vi "RichToFlatcif_channelcore_CreateFIFOInstanceResponse.vi"(5 "OutputClusterType":T1, 11 "InputCluster":T4) -> (3 "OutputCluster":T1)   [LabVIEW 2021, in "CIFCoreChannel_server.lvlib"]
uses:
  CIFCoreChannel_server.lvlib
  cif_channelcore_CreateFIFOInstanceResponse.ctl
  cif_channelcore_FIFOReference.ctl
  cif_common_Status.ctl
  cif_channelcore_CreateFIFOInstanceResponse_Flat.ctl
  cif_channelcore_FIFOReference_Flat.ctl
  cif_common_Status_Flat.ctl
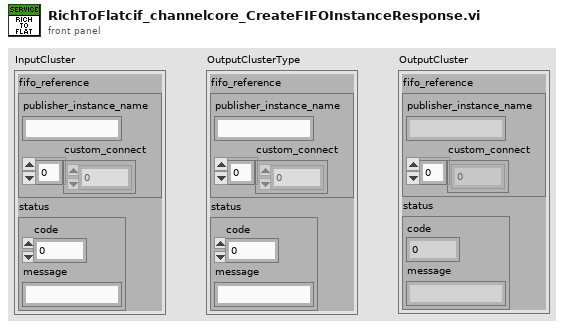
[diagram p1: front panel]
types:
  T1 = typedef "CIFCoreChannel_server.lvlib/cif_channelcore_CreateFIFOInstanceResponse_Flat.ctl" = cluster{"fifo_reference":T2, "status":T3}
  T2 = typedef "CIFCoreChannel_server.lvlib/cif_channelcore_FIFOReference_Flat.ctl" = cluster{"publisher_instance_name":string, "custom_connect":u8[]}
  T3 = typedef "CIFCoreChannel_server.lvlib/cif_common_Status_Flat.ctl" = cluster{"code":i32, "message":string}
  T4 = typedef "CIFCoreChannel_server.lvlib/cif_channelcore_CreateFIFOInstanceResponse.ctl" = cluster{"fifo_reference":T5, "status":T6}
  T5 = typedef "CIFCoreChannel_server.lvlib/cif_channelcore_FIFOReference.ctl" = cluster{"publisher_instance_name":string, "custom_connect":u8[]}
  T6 = typedef "CIFCoreChannel_server.lvlib/cif_common_Status.ctl" = cluster{"code":i32, "message":string}
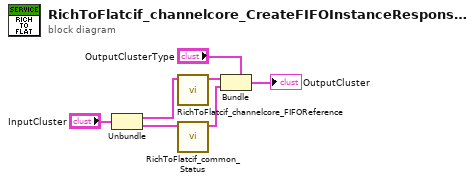
[diagram p0: block diagram]
diagram:
  n1 = Unbundle "Unbundle"("InputCluster") -> ("fifo_reference"=w4:T5, "status"=w2:T6)
  n2 = call "RichToFlatcif_channelcore_FIFOReference.vi"("InputCluster"=w4) -> ("OutputCluster"=w3:T2)  [unwired: 10 in]
  n3 = call "RichToFlatcif_common_Status.vi"("InputCluster"=w2) -> ("OutputCluster"=w1:T3)  [unwired: 10 in]
  n4 = Bundle "Bundle"(cluster="OutputClusterType", "fifo_reference"=w3, "status"=w1) -> (→"OutputCluster":T1)
